vi "Check For Solid or Full.vi"(8 "error in (no error)":errorcluster, 11 "Game Engine in":refnum<class "Game Engine.lvclass">) -> (0 "error out":errorcluster, 2 "Game Over":bool, 3 "Game Engine out":refnum<class "Game Engine.lvclass">)   [LabVIEW 2017, in "Game Engine.lvlib" / "Game Engine.lvclass"]
uses:
  Game Engine.lvclass
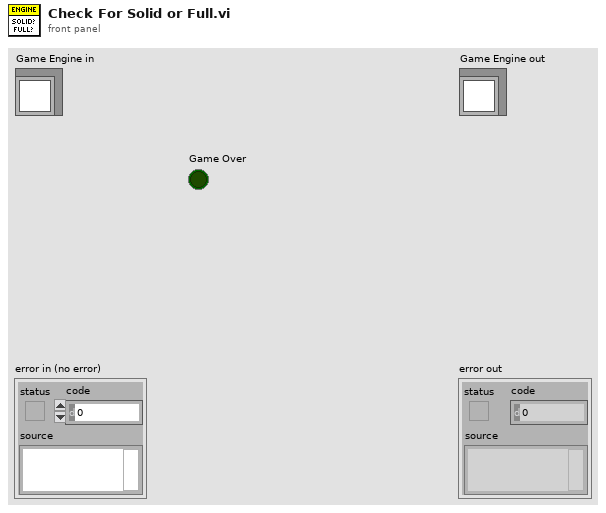
[diagram p1: front panel]
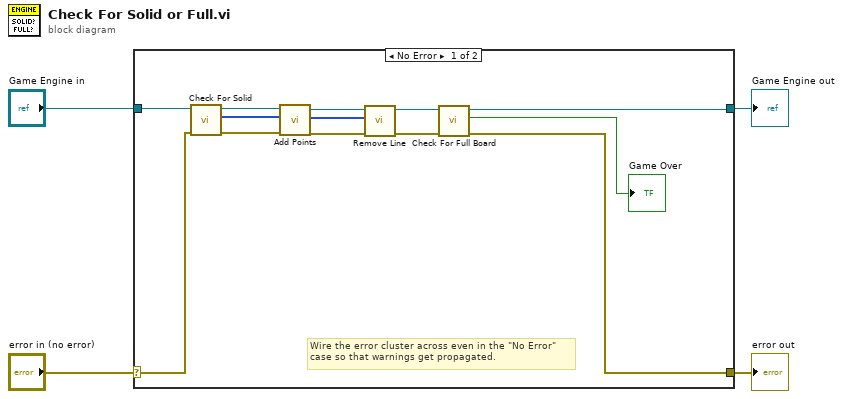
[diagram p0: block diagram]
diagram:
  n1 = case shown="No Error" "error in (no error)" {
    selector: "error in (no error)" -> [w6 w19]
    tunnel: [w5 w19] -> w3
    tunnel: [w7 w18] -> w1
    tunnel: "Game Engine in" -> [w17 w18]
    frame No Error {
      # "Wire the error cluster across even in the \"No Error\"\ncase so that warnings get propagated."
      n2 = call "Check For Solid.vi"("error in (no error)"=w6, "Game Engine in"=w17) -> ("error out"=w14:errorcluster, "Array"=w15:i32[], "Game Engine out"=w16:refnum<class "Game Engine.lvclass">)  [unwired: 7 in]
      n3 = call "Add Points.vi"("error in (no error)"=w14, "Solid Lines"=w15, "Game Engine in"=w16) -> ("error out"=w11:errorcluster, "Solid Lines (duplicate)"=w13:i32[], "Game Engine out"=w12:refnum<class "Game Engine.lvclass">)  [unwired: 6 in]
      n4 = call "Remove Line.vi"("error in (no error)"=w11, "Lines to Delete"=w13, "Game Engine in"=w12) -> ("error out"=w9:errorcluster, "Game Engine out"=w10:refnum<class "Game Engine.lvclass">)  [unwired: 7 in]
      n5 = call "Check For Full Board.vi"("error in (no error)"=w9, "Game Engine in"=w10) -> ("error out"=w5:errorcluster, "Pieces are Out of Bounds"=→"Game Over":bool, "Game Engine out"=w7:refnum<class "Game Engine.lvclass">)  [unwired: 7 in]
    }
    frame Error {
    }
  }
  "error out" <- w3
  "Game Engine out" <- w1
